vi "Sequence.FormatConditions.vi"(4 "Aliases.All":T3[](array[typedef]), 6 "Aliases Array":string[](array[string]), 8 "error in (no error)":errorcluster, 10 "Conditions":string[](array[string]), 11 "variant in":variant) -> (0 "error out":errorcluster, 1 "Warning":string, 2 "Condition":T1={"First Opreation"=enum."||", "Expression"=""}, 3 "variant out":variant)   [LabVIEW 2013, in "Simple Sequence Editor.lvlib"]
uses:
  Simple Sequence Editor.lvlib
  Types/ChannelProperties.ctl
  Types/Compiled.StepCondition.ctl
  Types/OperationTypes.ctl
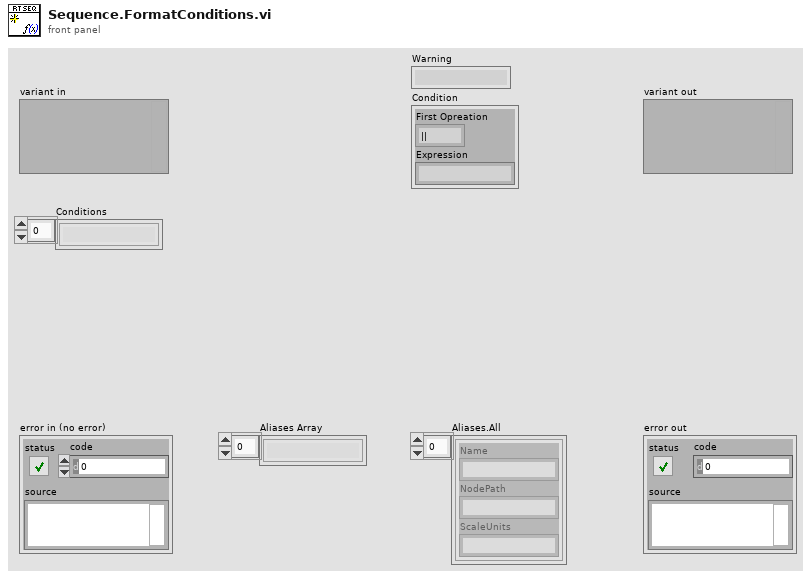
[diagram p1: front panel]
types:
  T1 = typedef "Simple Sequence Editor.lvlib/Compiled.StepCondition.ctl" = cluster{"First Opreation":T2, "Expression":string}
  T2 = typedef "Simple Sequence Editor.lvlib/OperationTypes.ctl" = enum8{"None", "&&", "||"}
  T3 = typedef "Simple Sequence Editor.lvlib/ChannelProperties.ctl" = cluster{"Name":string, "NodePath":string, "ScaleUnits":string}
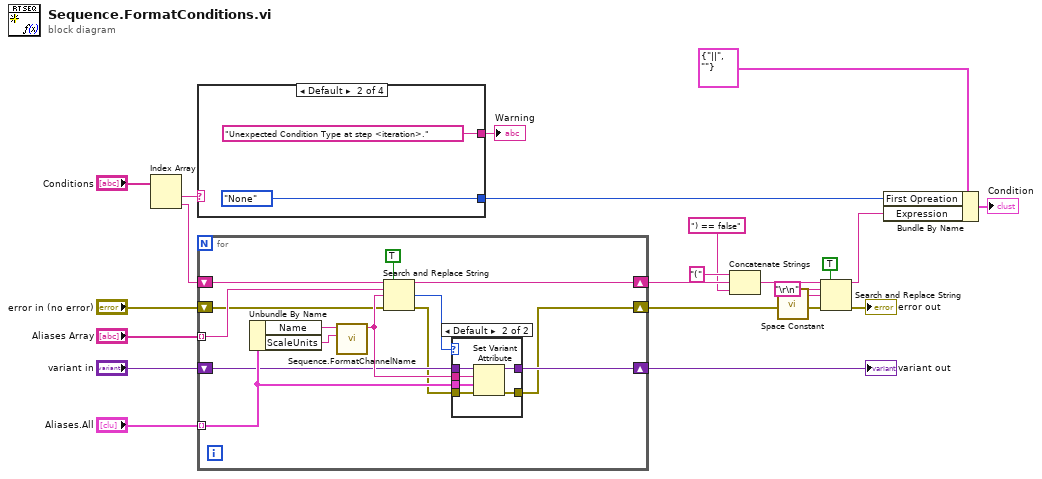
[diagram p0: block diagram]
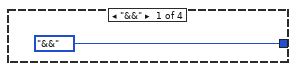
[diagram p3: hidden frame]
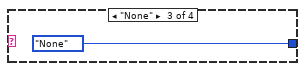
[diagram p4: hidden frame]
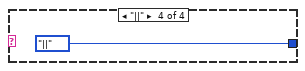
[diagram p5: hidden frame]
diagram:
  n1 = Index Array(array="Conditions") -> (element #1=w9:string, element #2=w8:string)  [unwired: 2 in]
  n2 = case shown="Default" w9 {
    tunnel: [OperationTypes."&&" OperationTypes."None" OperationTypes."None" OperationTypes."||"] -> w3
    tunnel: [_ "Unexpected Condition Type at step <iteration>." _ _] -> w5
    frame "&&" {
    }
    frame Default {
    }
    frame "None" {
    }
    frame "||" {
    }
  }
  "Warning" <- w5
  n3 = for {
    tunnel: "Aliases Array" -> [w41] mode=indexing
    tunnel: "Aliases.All" -> [w35] mode=indexing
    shift-right: [w28] -> w18
    shift-left: "error in (no error)" -> [w32]
    shift-right: [w36] -> w7
    shift-left: w8 -> [w40]
    shift-right: [w33] -> w22
    shift-left: "variant in" -> [w30]
    n4 = Unbundle By Name(w35) -> ("Name"=w38:string, "ScaleUnits"=w39:string)
    n5 = call "Sequence.FormatChannelName.vi"("ScaleUnits"=w39, "Name"=w38) -> ("ChannelName"=w34:string)  [unwired: 9 in]
    n6 = Search and Replace String(replace all?=TRUE ("replace all? (F)"), input string=w40, search string=w41, replace string=w34, error in=w32) -> (result string=w36:string, number of replacements=w31:i32, error out=w29:errorcluster)  [unwired: 3 in, 1 out]
    n7 = case shown="Default" w31 {
      tunnel: w35 -> [_ w49]
      tunnel: w34 -> [_ w48]
      tunnel: [w43 w47] -> w33
      tunnel: w30 -> [w43 w46]
      tunnel: w29 -> [w42 w45]
      tunnel: [w42 w44] -> w28
      frame -1, 0 {
      }
      frame Default {
        n8 = Set Variant Attribute(Variant=w46, name=w48, value=w49, error in=w45) -> (Variant out=w47:variant, error out=w44:errorcluster)  [unwired: 1 out]
      }
    }
  }
  "variant out" <- w22
  n9 = Concatenate Strings("(" ("string"), w7, ") == false" ("string")) -> (w15:string)
  n10 = call <vilib>:"Space Constant.vi"() -> ("String"=w17:string)
  n11 = Search and Replace String(replace all?=TRUE ("replace all? (F)"), input string=w15, search string="\r\n", replace string=w17, error in=w18) -> (result string=w2:string, error out=→"error out":errorcluster)  [unwired: 3 in, 2 out]
  n12 = Bundle By Name(cluster=T1 {"First Opreation"=enum."||", "Expression"=""} ("Condition"), "First Opreation"=w3, "Expression"=w2) -> (→"Condition":T1)
